vi "SetValves.vi"(8 "Boolean Array":bool[](array[boolean]), 11 "Indices":i32[](array[numeric])) -> ()   [LabVIEW 2011]
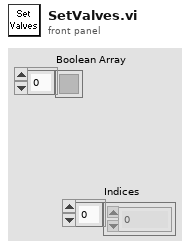
[diagram p1: front panel]
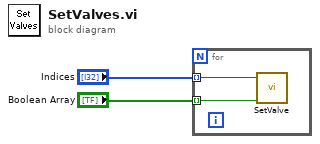
[diagram p0: block diagram]
diagram:
  n1 = for {
    tunnel: "Indices" -> [w4] mode=indexing
    tunnel: "Boolean Array" -> [w3] mode=indexing
    n2 = call "SetValve.vi"("Open/Close"=w3, "Valve"=w4) -> ()  [unwired: 10 in]
  }
